vi "Find LVLIBP Member.vi"(8 "error in (no error)":errorcluster, 10 "Member Name":string, 11 "LVLIBP Parser in":refnum<class "LVLIBP Parser.lvclass">) -> (0 "error out":errorcluster, 1 "Found ?":bool, 2 "path":path, 3 "LVLIBP Parser out":refnum<class "LVLIBP Parser.lvclass">)   [LabVIEW 2018, in ".LVLIBP CD XML Updater.lvlib" / "LVLIBP Parser.lvclass"]
uses:
  LVLIBP Parser.lvclass
  LVLIBP Parser.lvclass/LVLIBP Parser.ctl
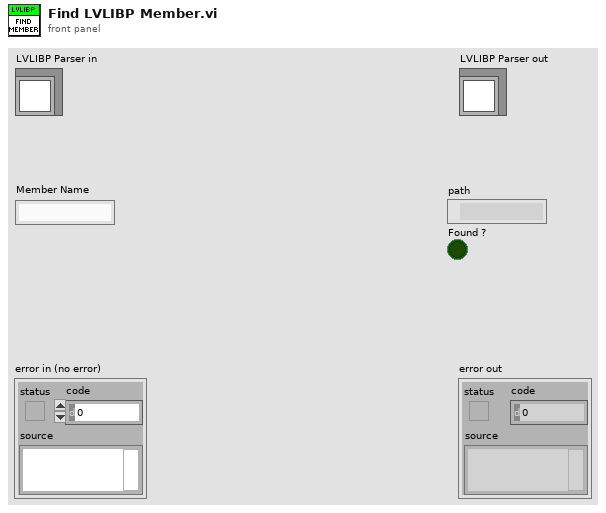
[diagram p1: front panel]
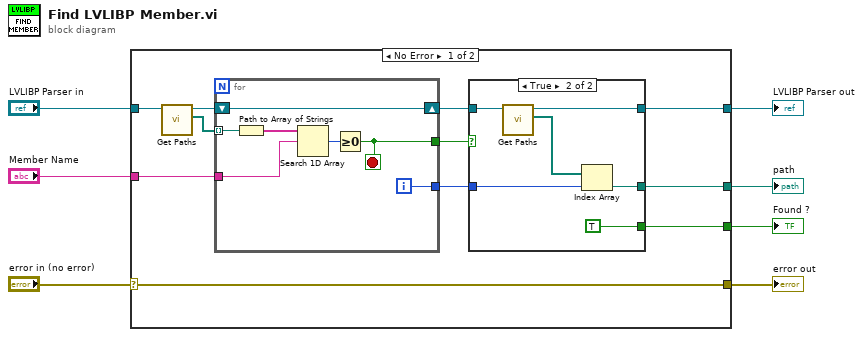
[diagram p0: block diagram]
diagram:
  n1 = case shown="No Error" "error in (no error)" {
    selector: "error in (no error)" -> [w18 w34]
    tunnel: [w18 w34] -> w6
    tunnel: [w13 w33] -> w4
    tunnel: "LVLIBP Parser in" -> [w10 w33]
    tunnel: "Member Name" -> [w17 _]
    tunnel: [w12 _] -> w2
    tunnel: [w11 _] -> w1
    frame No Error {
      n2 = call "Get Paths.vi"("LVLIBP Parser in"=w10) -> ("Paths"=w8:path[], "LVLIBP Parser out"=w9:refnum<class "LVLIBP Parser.lvclass">)  [unwired: 9 in]
      n3 = for {
        tunnel: w17 -> [w27]
        shift-right: [w32] -> w15
        shift-left: w9 -> [w32]
        tunnel: [w31] -> w16
        tunnel: [w30] -> w14
        tunnel: w8 -> [w29] mode=indexing
        i -> [w30]
        stop <- w31 stop-if-true
        n4 = Path to Array of Strings(0:w29) -> (2:w28:string[])  [unwired: 1 out]
        n5 = Search 1D Array(1D array=w28, element=w27) -> (index of element=w26:i32)  [unwired: 1 in]
        n6 = Greater Or Equal To 0?(x=w26) -> (x >= 0?=w31:bool)
      }
      n7 = case shown="True" w16 {
        tunnel: w15 -> [w19 w25]
        tunnel: [w19 w24] -> w13
        tunnel: w14 -> [_ w22]
        tunnel: [_ w21] -> w12
        tunnel: [_ TRUE] -> w11
        frame False {
        }
        frame True {
          n8 = call "Get Paths.vi"("LVLIBP Parser in"=w25) -> ("Paths"=w23:path[], "LVLIBP Parser out"=w24:refnum<class "LVLIBP Parser.lvclass">)  [unwired: 9 in]
          n9 = Index Array(array=w23, index=w22) -> (element=w21:path)
        }
      }
    }
    frame Error {
    }
  }
  "error out" <- w6
  "LVLIBP Parser out" <- w4
  "path" <- w2
  "Found ?" <- w1
